vi "Read (Math).vi"(8 "error in (no error)":errorcluster, 10 "Reset After Read (False)":bool, 11 "VISA resource name":refnum<visa-resource-name>) -> (0 "error out":errorcluster, 1 "Count":dbl, 2 "Average":dbl, 3 "VISA resource name out":refnum<visa-resource-name>, 5 "Minimum":dbl, 7 "Maximum":dbl)   [LabVIEW 2014, in "Fluke 884X Series.lvlib"]
doc: "Read (Math) returns the minimum, maximum, average, and count values from multiple measurements. This VI requires that Min/Max is set in Configure Math and should be called after multiple measurements have been taken."
uses:
  Fluke 884X Series.lvlib
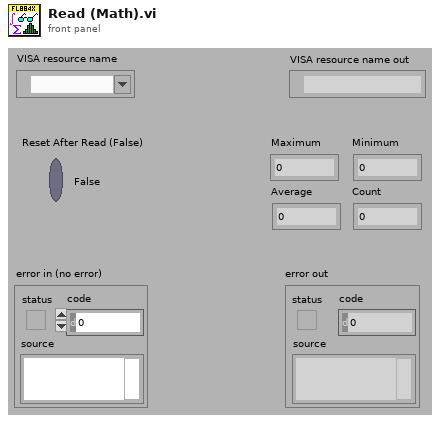
[diagram p1: front panel]
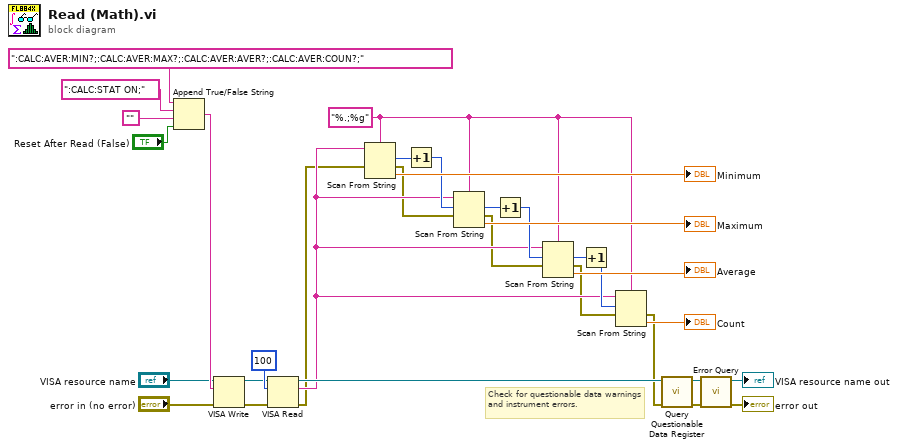
[diagram p0: block diagram]
diagram:
  w8 = "%.;%g" ("format string")
  # "Check for questionable data warnings and instrument errors."
  n1 = Append True/False String(1:"Reset After Read (False)", 2:"" ("Empty String Constant"), 3:":CALC:STAT ON;", 4:":CALC:AVER:MIN?;:CALC:AVER:MAX?;:CALC:AVER:AVER?;:CALC:AVER:COUN?;") -> (0:w18:string)
  n2 = VISA Write(VISA resource name="VISA resource name", write buffer=w18, error in (no error)="error in (no error)") -> (VISA resource name out=w15:refnum<visa-resource-name>, error out=w16:errorcluster)  [unwired: 1 out]
  n3 = VISA Read(VISA resource name=w15, byte count=u32 100, error in (no error)=w16) -> (VISA resource name out=w23:refnum<visa-resource-name>, read buffer=w7:string, error out=w6:errorcluster)  [unwired: 1 out]
  n4 = Scan From String(format string=w8, input string=w7, error in=w6) -> (offset past scan=w9:u32, error out=w5:errorcluster, output 1=→"Minimum":dbl)  [unwired: 2 in, 1 out]
  n5 = Increment(x=w9) -> (x+1=w10:u32)
  n6 = Scan From String(format string=w8, input string=w7, initial scan location=w10, error in=w5) -> (offset past scan=w11:u32, error out=w4:errorcluster, output 1=→"Maximum":dbl)  [unwired: 1 in, 1 out]
  n7 = Increment(x=w11) -> (x+1=w12:u32)
  n8 = Scan From String(format string=w8, input string=w7, initial scan location=w12, error in=w4) -> (offset past scan=w13:u32, error out=w3:errorcluster, output 1=→"Average":dbl)  [unwired: 1 in, 1 out]
  n9 = Increment(x=w13) -> (x+1=w14:u32)
  n10 = Scan From String(format string=w8, input string=w7, initial scan location=w14, error in=w3) -> (error out=w22:errorcluster, output 1=→"Count":dbl)  [unwired: 1 in, 2 out]
  n11 = call "Query Questionable Data Register.vi"("error in (no error)"=w22, "VISA resource name"=w23) -> ("error out"=w25:errorcluster, "VISA resource name out"=w24:refnum<visa-resource-name>)  [unwired: 7 in, 1 out]
  n12 = call "Error Query.vi"("error in (no error)"=w25, "VISA resource name"=w24) -> ("error out"=→"error out":errorcluster, "VISA resource name out"=→"VISA resource name out":refnum<visa-resource-name>)  [unwired: 6 in, 2 out]
